vi "Vision Inspection Example (For Exe Application).vi"(4 "Thread No.":u32, 5 "ProgramRef":refnum<vi>, 6 "Thread Mod Recive":refnum<queue>[](array[refnum]), 7 "ThreadsQueue":refnum<queue>[](array[refnum]), 8 "ThreadInfoIN":T3, 10 "StackIn":cluster{"Program":i32, "Prog Index":i32}[](array[cluster]), 11 "PrameterS":string) -> (0 "ThreadInfoOUT":T3, 2 "StackOut":cluster{"Program":i32, "Prog Index":i32}[](array[cluster]), 3 "ErrorCode":string)   [LabVIEW 2020]
uses:
  <vilib>/vision/NI_Vision_Development_Module.lvlib
panel:
  in  "SettingAbort":bool
  out "P2":T1(plugin-control)
  out "P1":T1(plugin-control)
  out "Update?":bool
  in  "SettingDone":bool
  out "Result":sgl
  in  "OP Overwrite":string(combo)
  in  "SettingData":T2={"MatchParameters"={"Number of Matches Requested"=1, "Minimum Match Score"=600.0, "Angle Ranges"=[{"Start Angle"=0.0, "End Angle"=360.0}]}, "Algorithm"=1, "Pattern1ImageStriing"="", "Pattern1"={"x"=2703.5, "y"=1250.0}, "ROI"={"Global Rectangle"=[816, 381, 3234, 2692], "Contours"=[{"Contour Type"=0, "ROI Type"=3, "Points"=[816, 381, 3234, 2692]}, {"Contour Type"=0, "ROI Type"=3, "Points"=[2426, 953, 2982, 1548]}, {"Contour Type"=0, "ROI Type"=3, "Points"=[1311, 1495, 1906, 2113]}]}, "Range"={"Minimum"=160.0, "Maximum"=180.0}, "Pattern2ImageStriing"="", "Pattern2"={"x"=1608.0, "y"=1803.5}, "PatternAngle"=153.19487, "PatternImageStriing"=""} {"Pattern2"."y" format="%.2f"; "Pattern2"."x" format="%.2f"; "Range"."Maximum" format="%.2f"; "Range"."Minimum" format="%.2f"; "Pattern1"."y" format="%.2f"; "Pattern1"."x" format="%.2f"; "Algorithm" items=["All", "Low Discrepancy Sampling", "Grayscale Value Pyramid", "Gradients Pyramid"]}
  in  "ImagePath":path=path "D:/Project/Z-Other/Boash2M/sample02 cover black.png"
  out "Test":T1(plugin-control)
  out "FindPattern1?":bool
  in  "IMAQ?":bool=TRUE
  out "FindPattern2?":bool
  out "SampleAngle":sgl
  out "Pattern":T1(plugin-control)
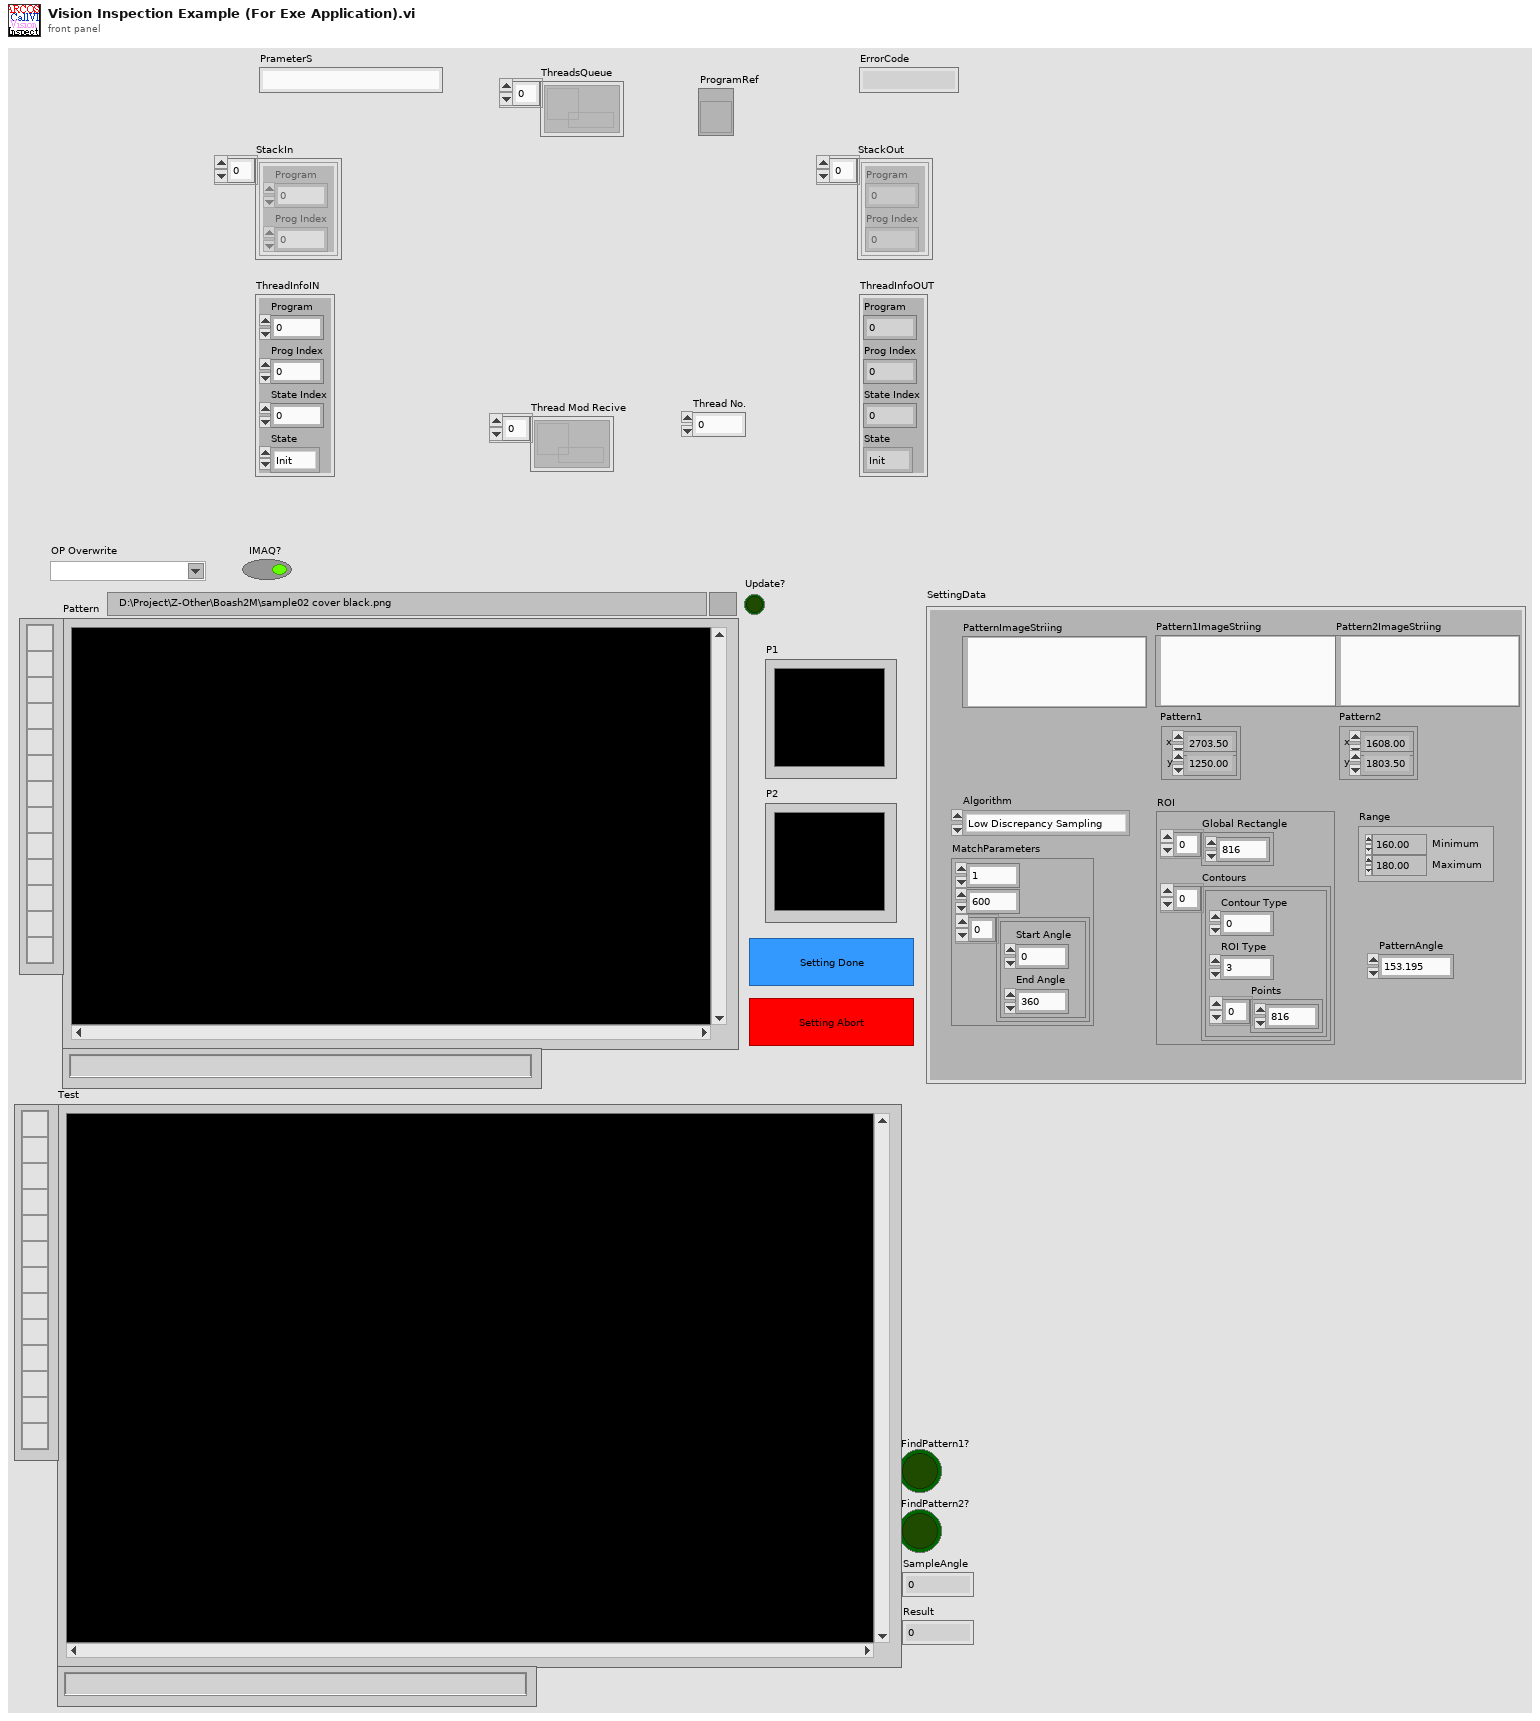
[diagram p1: front panel]
types:
  T1 = typedef "IMAQ Image.ctl" = refnum<image>
  T2 = cluster{"MatchParameters":cluster{"Number of Matches Requested":i32, "Minimum Match Score":sgl, "Angle Ranges":cluster{"Start Angle":sgl, "End Angle":sgl}[]}, "Algorithm":i32, "Pattern1ImageStriing":string, "Pattern1":cluster{"x":sgl, "y":sgl}, "ROI":cluster{"Global Rectangle":i32[], "Contours":cluster{"Contour Type":u32, "ROI Type":u32, "Points":i32[]}[]}, "Range":cluster{"Minimum":sgl, "Maximum":sgl}, "Pattern2ImageStriing":string, "Pattern2":cluster{"x":sgl, "y":sgl}, "PatternAngle":sgl, "PatternImageStriing":string}
  T3 = cluster{"Program":i32, "Prog Index":i32, "State Index":i32, "State":enum16{"Init", "Idle", "Auto Start", "Auto Running", "Step Start", "Step Running", "Suspend", "Restart", "Stop", "Reset"}}
  T4 = typedef "Image Type" = u32
  T5 = cluster{"Global Rectangle":i32[], "Contours":cluster{"Contour Type":u32, "ROI Type":u32, "Points":i32[]}[]}
  T6 = cluster{"Contour Type":u32, "ROI Type":u32, "Points":i32[]}[]
  T7 = cluster{"Contour Type":u32, "ROI Type":u32, "Points":i32[]}
  T8 = enum16{"Init", "Idle", "Auto Start", "Auto Running", "Step Start", "Step Running", "Suspend", "Restart", "Stop", "Reset"}
  T9 = cluster{"Number of Matches Requested":i32, "Minimum Match Score":sgl, "Angle Ranges":cluster{"Start Angle":sgl, "End Angle":sgl}[]}
  T10 = cluster{"Position":cluster{"x":sgl, "y":sgl}, "Angle":sgl, "Scale":sgl, "Score":sgl, "Bounding Box":cluster{"x":sgl, "y":sgl}[]}[]
  T11 = cluster{"Position":cluster{"x":sgl, "y":sgl}, "Angle":sgl, "Scale":sgl, "Score":sgl, "Bounding Box":cluster{"x":sgl, "y":sgl}[]}
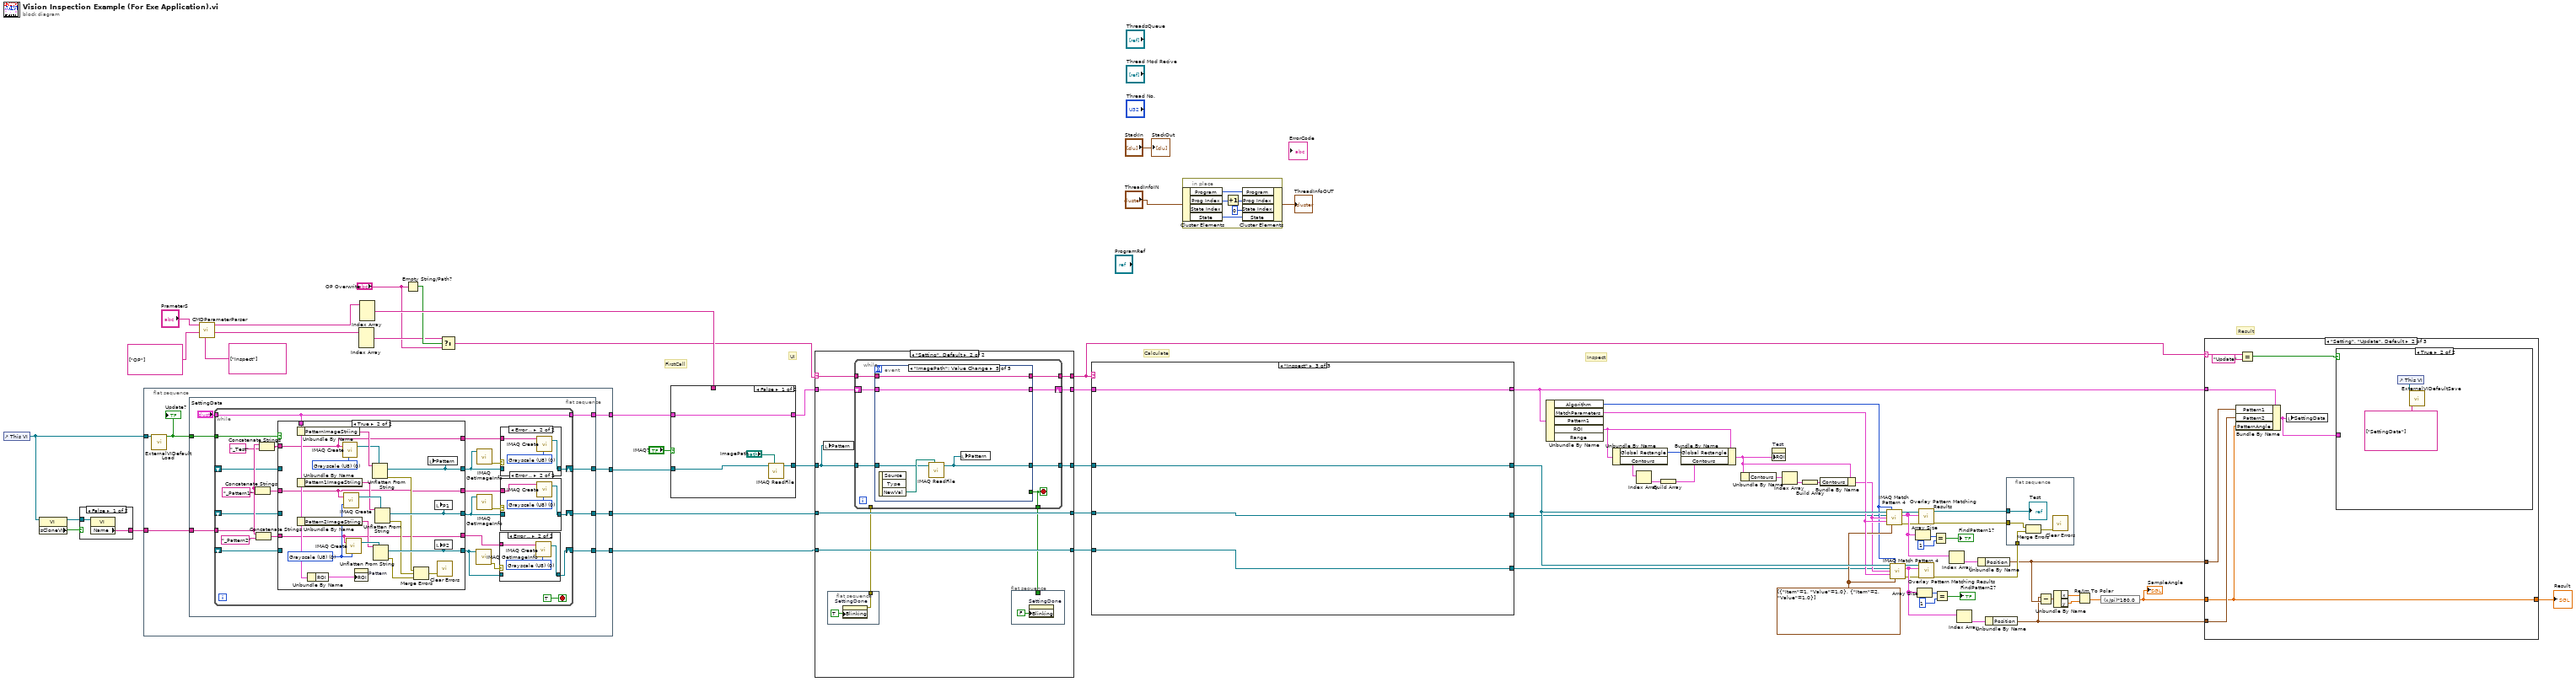
[diagram p0: block diagram]
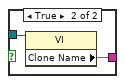
[diagram p2: hidden frame]
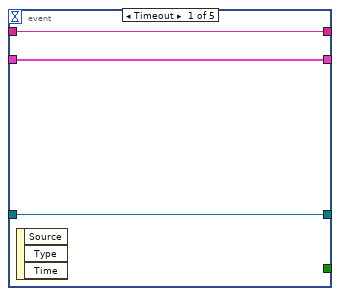
[diagram p8: hidden frame]
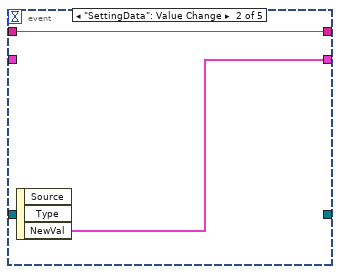
[diagram p9: hidden frame]
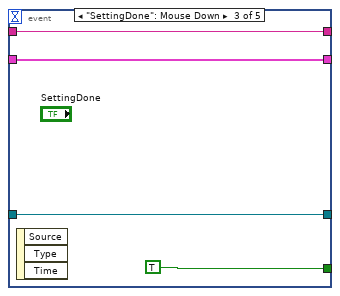
[diagram p10: hidden frame]
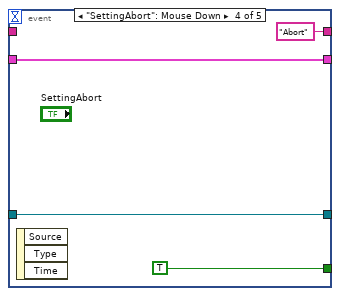
[diagram p11: hidden frame]
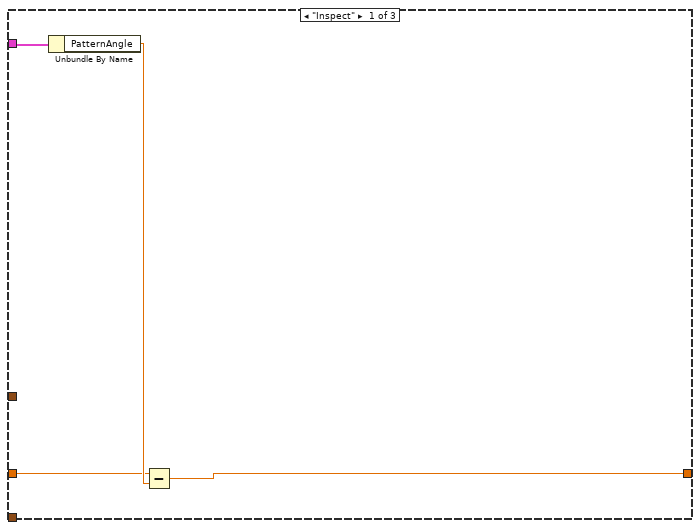
[diagram p12: hidden frame]
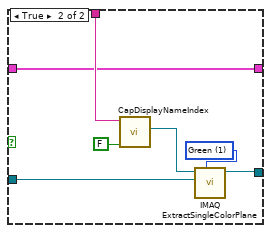
[diagram p15: hidden frame]
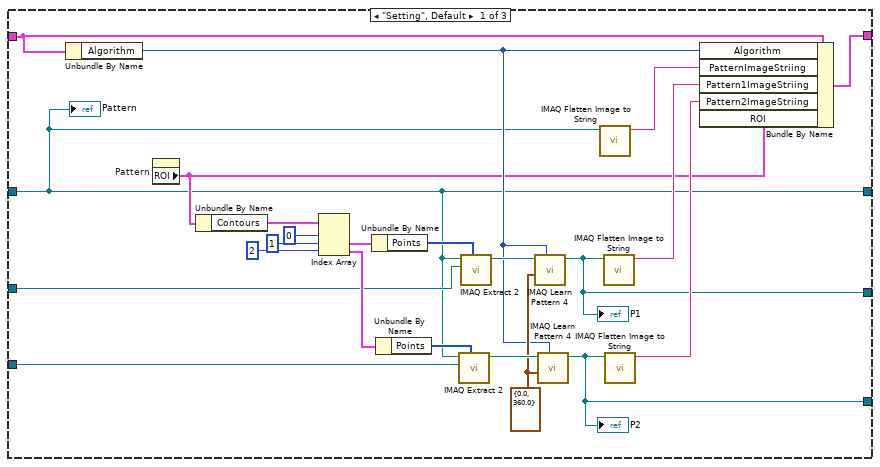
[diagram p16: hidden frame]
diagram:
  w37 = cluster{"Item":u16, "Value":dbl}[] [{"Item"=1, "Value"=1.0}, {"Item"=2, "Value"=1.0}] ("Advanced Options")
  # "Result"
  # "Inspect"
  # "Calculate"
  # "FirstCall"
  # "UI"
  n1 = control-ref of="This VI"() -> (w14:refnum<vi>)
  n2 = property class="VI"(reference=w14) -> (reference out=w15:refnum<vi>, "IsCloneVI"=w16:bool)  [unwired: 1 in, 1 out]
  n3 = case shown="False" w16 {
    tunnel: w15 -> [w73 w75]
    tunnel: [w72 w74] -> w2
    frame False {
      n4 = property class="VI"(reference=w73) -> ("Name"=w72:string)  [unwired: 1 in, 2 out]
    }
    frame True {
      n5 = property class="VI"(reference=w75) -> ("Clone Name"=w74:string)  [unwired: 1 in, 2 out]
    }
  }
  n6 = flat-sequence {
    tunnel: [w82] -> w18
    tunnel: w14 -> [w80]
    tunnel: [w77] -> w4
    tunnel: [w76] -> w3
    tunnel: w2 -> [w79]
    tunnel: [w78] -> w1
    frame #0 {
      n7 = call "ExternalVIDefaultLoad.vi"("VI in"=w80) -> ("Update?"=w81:bool)  [unwired: 10 in]
      "Update?" <- w81
      n8 = flat-sequence {
        tunnel: [w88] -> w82
        tunnel: w81 -> [w87]
        tunnel: w79 -> [w86]
        tunnel: [w85] -> w78
        tunnel: [w84] -> w77
        tunnel: [w83] -> w76
        frame #0 {
          n9 = while {
            shift-right: [w98] -> w85
            shift-left: _ -> [w111]
            shift-right: [w96] -> w84
            shift-left: _ -> [w110]
            shift-right: [w90] -> w83
            shift-left: _ -> [w109]
            tunnel: "SettingData" -> [w108]
            tunnel: [w108] -> w88
            tunnel: w87 -> [w113]
            tunnel: w86 -> [w112]
            stop <- TRUE stop-if-true
            n10 = Concatenate Strings(w112, "_Pattern1" ("string")) -> (w104:string)
            n11 = Concatenate Strings(w112, "_Pattern2" ("string")) -> (w102:string)
            n12 = Concatenate Strings(w112, "_Test" ("string")) -> (w106:string)
            n13 = case shown="True" w113 {
              tunnel: w111 -> [w130 _]
              tunnel: w110 -> [w132 _]
              tunnel: w109 -> [w131 _]
              tunnel: w108 -> [_ w145]
              tunnel: [w130 w142] -> w99
              tunnel: [w132 w141] -> w94
              tunnel: [w131 w140] -> w92
              tunnel: w106 -> [w129 w134]
              tunnel: w104 -> [w128 w135]
              tunnel: w102 -> [w127 w133]
              tunnel: [w128 w135] -> w95
              tunnel: [w129 w134] -> w100
              tunnel: [w127 w133] -> w91
              frame False {
              }
              frame True {
                w152 = T4 0 items=["Grayscale (U8)", "Grayscale (I16)", "Grayscale (SGL)", "Complex (CSG)", "RGB (U32)", "HSL (U32)", "RGB (U64)", "Grayscale (U16)"] ("Image Type")
                w143 = T4 0 items=["Grayscale (U8)", "Grayscale (I16)", "Grayscale (SGL)", "Complex (CSG)", "RGB (U32)", "HSL (U32)", "RGB (U64)", "Grayscale (U16)"] ("Image Type")
                n14 = Unbundle By Name(w145) -> ("PatternImageStriing"=w151:string)
                n15 = Unbundle By Name(w145) -> ("Pattern1ImageStriing"=w147:string)
                n16 = Unbundle By Name(w145) -> ("Pattern2ImageStriing"=w146:string)
                n17 = Unbundle By Name(w145) -> ("ROI"=w144:T5)
                n18 = call "IMAQ Create"("Image Name"=w134, "Image Type"=w152) -> ("New Image"=w150:T1)  [unwired: 3 in, 1 out]
                n19 = call "IMAQ Create"("Image Name"=w135, "Image Type"=w143) -> ("New Image"=w149:T1)  [unwired: 3 in, 1 out]
                n20 = call "IMAQ Create"("Image Name"=w133, "Image Type"=w143) -> ("New Image"=w148:T1)  [unwired: 3 in, 1 out]
                n21 = property on="Pattern" class="ImageControl"("ROI"=w144) -> ()  [unwired: 2 in, 2 out]
                n22 = Unflatten From String(type=w150, binary string=w151) -> (value=w142:T1, error out=w139:errorcluster)  [unwired: 3 in, 1 out]
                n23 = Unflatten From String(type=w148, binary string=w146) -> (value=w140:T1, error out=w137:errorcluster)  [unwired: 3 in, 1 out]
                n24 = Unflatten From String(type=w149, binary string=w147) -> (value=w141:T1, error out=w138:errorcluster)  [unwired: 3 in, 1 out]
                n25 = Merge Errors(w139, w138, w137) -> (w136:errorcluster)
                n26 = local write "Pattern"(w142) -> ()
                n27 = local write "P1"(w141) -> ()
                n28 = local write "P2"(w140) -> ()
                n29 = call <vilib>:"Clear Errors.vi"("error in (no error)"=w136) -> ()  [unwired: 5 in, 2 out]
              }
            }
            n30 = call "IMAQ GetImageInfo"("Image"=w92) -> ("error out"=w93:errorcluster)  [unwired: 3 in, 7 out]
            n31 = call "IMAQ GetImageInfo"("Image"=w99) -> ("error out"=w101:errorcluster)  [unwired: 3 in, 7 out]
            n32 = call "IMAQ GetImageInfo"("Image"=w94) -> ("error out"=w97:errorcluster)  [unwired: 3 in, 7 out]
            n33 = case shown="Error .." w93 {
              tunnel: w91 -> [_ w118]
              tunnel: w92 -> [w115 _]
              tunnel: [w115 w116] -> w90
              frame No Error {
              }
              frame Error {
                w117 = T4 0 items=["Grayscale (U8)", "Grayscale (I16)", "Grayscale (SGL)", "Complex (CSG)", "RGB (U32)", "HSL (U32)", "RGB (U64)", "Grayscale (U16)"] ("Image Type")
                n34 = call "IMAQ Create"("Image Name"=w118, "Image Type"=w117) -> ("New Image"=w116:T1)  [unwired: 3 in, 1 out]
              }
            }
            n35 = case shown="Error .." w101 {
              tunnel: w100 -> [_ w126]
              tunnel: w99 -> [w123 _]
              tunnel: [w123 w124] -> w98
              frame No Error {
              }
              frame Error {
                w125 = T4 0 items=["Grayscale (U8)", "Grayscale (I16)", "Grayscale (SGL)", "Complex (CSG)", "RGB (U32)", "HSL (U32)", "RGB (U64)", "Grayscale (U16)"] ("Image Type")
                n36 = call "IMAQ Create"("Image Name"=w126, "Image Type"=w125) -> ("New Image"=w124:T1)  [unwired: 3 in, 1 out]
              }
            }
            n37 = case shown="Error .." w97 {
              tunnel: w94 -> [w119 _]
              tunnel: [w119 w121] -> w96
              tunnel: w95 -> [_ w120]
              frame No Error {
              }
              frame Error {
                w122 = T4 0 items=["Grayscale (U8)", "Grayscale (I16)", "Grayscale (SGL)", "Complex (CSG)", "RGB (U32)", "HSL (U32)", "RGB (U64)", "Grayscale (U16)"] ("Image Type")
                n38 = call "IMAQ Create"("Image Name"=w120, "Image Type"=w122) -> ("New Image"=w121:T1)  [unwired: 3 in, 1 out]
              }
            }
          }
        }
      }
    }
  }
  n39 = call "CMDParameterParser.vi"("DeafultValues"=string[] ["Inspect"], "RequiredKeys"=string[] ["OP"], "CMDParameter"="PrameterS") -> ("KeyValues"=w67:string[], "Input"=w65:string[])  [unwired: 6 in, 1 out]
  n40 = Index Array(array=w67) -> (element #1=w29:string)  [unwired: 3 in, 2 out]
  n41 = Index Array(array=w65) -> (element #1=w64:string)  [unwired: 3 in, 2 out]
  n42 = Empty String/Path?(string/path="OP Overwrite") -> (empty?=w30:bool)
  n43 = Select(t=w29, s=w30, f="OP Overwrite") -> (s? t:f=w13:string)
  n44 = case shown="False" "IMAQ?" {
    tunnel: [w156 w159] -> w19
    tunnel: w64 -> [_ w162]
    tunnel: w1 -> [w154 w158]
    tunnel: w18 -> [w153 w157]
    tunnel: [w153 w157] -> w17
    frame False {
      n45 = call "IMAQ ReadFile"("File Path"="ImagePath", "Image"=w154) -> ("Image Out"=w156:T1)  [unwired: 5 in, 4 out]
    }
    frame True {
      w161 = 1 items=["Red", "Green", "Blue", "Hue", "Saturation", "Luminance", "Value", "Intensity"] ("Color Plane")
      n46 = call "CapDisplayNameIndex.vi"("Init?"=FALSE, "CamName"=w162) -> ("IMAQ"=w160:T1)  [unwired: 3 in, 3 out]
      n47 = call "IMAQ ExtractSingleColorPlane"("Color Plane"=w161, "Image Dst"=w158, "Image Src"=w160) -> ("Image Dst Out"=w159:T1)  [unwired: 7 in, 1 out]
    }
  }
  n48 = case shown="\"Setting\", Default" w13 {
    selector: w13 -> [w164 w171]
    tunnel: w17 -> [w168 w175]
    tunnel: [w168 w174] -> w22
    tunnel: w19 -> [w167 w169]
    tunnel: [w167 w176] -> w21
    tunnel: w4 -> [w166 w178]
    tunnel: [w166 w178] -> w20
    tunnel: w3 -> [w165 w177]
    tunnel: [w165 w177] -> w9
    tunnel: [w164 w170] -> w12
    frame "Inspect" {
    }
    frame "Setting", Default {
      n49 = local write "Pattern"(w169) -> ()
      n50 = flat-sequence {
        tunnel: [w180] -> w173
        frame #0 {
          n51 = property on="SettingDone" class="Bool"("Blinking"=TRUE) -> (error out=w180:errorcluster)  [unwired: 2 in, 1 out]
        }
      }
      n52 = while {
        tunnel: w169 -> [w188]
        tunnel: [w187] -> w176
        shift-right: [w186] -> w174
        shift-left: w175 -> [w185]
        tunnel: w173 -> [_]
        tunnel: [w184] -> w172
        tunnel: w171 -> [w183]
        tunnel: [w182] -> w170
        stop <- w184 stop-if-true
        n53 = event shown="[4] \"ImagePath\": Value Change" {
          selector: _ -> [_ _ _ _ _]
          dyn-events: _ -> [_ _ _ _ _]
          timeout: _ -> [_ _ _ _ _]
          tunnel: [_ _ TRUE TRUE _] -> w184
          tunnel: w188 -> [w191 _ w196 w200 w205]
          tunnel: [w191 _ w196 w200 w203] -> w187
          tunnel: [w189 w193 w195 w199 w204] -> w186
          tunnel: w185 -> [w189 _ w195 w199 w204]
          tunnel: w183 -> [w190 w192 w194 _ w202]
          tunnel: [w190 w192 w194 "Abort" w202] -> w182
          event Timeout {
            n54 = event-data() -> ()  [unwired: 1 in, 3 out]
          }
          event "SettingData": Value Change {
            n55 = event-data() -> ("NewVal"=w193:T2)  [unwired: 1 in, 2 out]
          }
          event "SettingDone": Mouse Down {
            n56 = event-data() -> ()  [unwired: 1 in, 3 out]
          }
          event "SettingAbort": Mouse Down {
            n57 = event-data() -> ()  [unwired: 1 in, 3 out]
          }
          event "ImagePath": Value Change {
            n58 = event-data() -> ("NewVal"=w206:path)  [unwired: 1 in, 2 out]
            n59 = call "IMAQ ReadFile"("File Path"=w206, "Image"=w205) -> ("Image Out"=w203:T1)  [unwired: 5 in, 4 out]
            n60 = local write "Pattern"(w203) -> ()
          }
        }
      }
      n61 = flat-sequence {
        tunnel: w172 -> [_]
        frame #0 {
          n62 = property on="SettingDone" class="Bool"("Blinking"=FALSE) -> ()  [unwired: 2 in, 2 out]
        }
      }
    }
  }
  n63 = case shown="\"Inspect\"" w12 {
    tunnel: w22 -> [w215 w233 w236]
    tunnel: w21 -> [w208 w232 w237]
    tunnel: [w214 w233 w236] -> w31
    tunnel: [w210 w231 w235] -> w6
    tunnel: [w209 w230 w234] -> w5
    tunnel: [w208 w232 w237] -> w39
    tunnel: w9 -> [w211 w230 w234]
    tunnel: w20 -> [w212 w231 w235]
    frame "Setting", Default {
      w218 = cluster{"Start Angle":sgl, "End Angle":sgl} {"Start Angle"=0.0, "End Angle"=360.0} ("Angle Range")
      n64 = Unbundle By Name(w215) -> ("Algorithm"=w216:i32)
      n65 = property on="Pattern" class="ImageControl"() -> ("ROI"=w213:T5)  [unwired: 2 in, 2 out]
      n66 = Unbundle By Name(w213) -> ("Contours"=w228:T6)
      n67 = Index Array(array=w228, index #1=0 ("index"), index #2=1 ("index"), index #3=2 ("index")) -> (element #2=w223:T7, element #3=w220:T7)  [unwired: 1 out]
      n68 = Unbundle By Name(w223) -> ("Points"=w222:i32[])
      n69 = Unbundle By Name(w220) -> ("Points"=w221:i32[])
      n70 = call "IMAQ Extract 2"("Optional Rectangle"=w221, "Image Dst"=w211, "Image Src"=w208) -> ("Image Dst Out"=w219:T1)  [unwired: 7 in, 1 out]
      n71 = call "IMAQ Extract 2"("Optional Rectangle"=w222, "Image Dst"=w212, "Image Src"=w208) -> ("Image Dst Out"=w226:T1)  [unwired: 7 in, 1 out]
      n72 = call "IMAQ Learn Pattern 4"("Algorithm"=w216, "Angle Range"=w218, "Image"=w226) -> ("Template Image Out"=w210:T1)  [unwired: 6 in, 2 out]
      "P1" <- w210
      n73 = call "IMAQ Learn Pattern 4"("Algorithm"=w216, "Angle Range"=w218, "Image"=w219) -> ("Template Image Out"=w209:T1)  [unwired: 6 in, 2 out]
      "P2" <- w209
      n74 = call "IMAQ Flatten Image to String"("Image"=w208) -> ("Data String"=w207:string)  [unwired: 9 in, 1 out]
      n75 = call "IMAQ Flatten Image to String"("Image"=w210) -> ("Data String"=w229:string)  [unwired: 9 in, 1 out]
      n76 = call "IMAQ Flatten Image to String"("Image"=w209) -> ("Data String"=w217:string)  [unwired: 9 in, 1 out]
      n77 = Bundle By Name(cluster=w215, "Algorithm"=w216, "PatternImageStriing"=w207, "Pattern1ImageStriing"=w229, "Pattern2ImageStriing"=w217, "ROI"=w213) -> (w214:T2)
      "Pattern" <- w208
    }
    frame "Abort" {
    }
    frame "Inspect" {
    }
  }
  n78 = in-place {
    n79 = in-place-cluster #1("ThreadInfoIN") -> ("Program"=w242:i32, "Prog Index"=w240:i32, "State"=w238:T8)  [unwired: 1 out]
    n80 = Increment(x=w240) -> (x+1=w241:i32)
    n81 = in-place-cluster #1("Program"=w242, "Prog Index"=w241, "State Index"=0, "State"=w238) -> (→"ThreadInfoOUT":T3)
  }
  n82 = Unbundle By Name(w31) -> ("Algorithm"=w32:i32, "MatchParameters"=w38:T9, "ROI"=w48:T5)  [unwired: 2 out]
  n83 = Unbundle By Name(w48) -> ("Global Rectangle"=w47:i32[], "Contours"=w44:T6)
  n84 = Index Array(array=w44) -> (element=w45:T7)  [unwired: 1 in]
  n85 = Build Array(w45) -> (w46:T6)
  n86 = Bundle By Name(cluster=w48, "Global Rectangle"=w47, "Contours"=w46) -> (w40:T5)
  n87 = Unbundle By Name(w40) -> ("Contours"=w50:T6)
  n88 = property on="Test" class="ImageControl"("ROI"=w40) -> ()  [unwired: 2 in, 2 out]
  n89 = Index Array(array=w50) -> (element=w51:T7)  [unwired: 1 in]
  n90 = Build Array(w51) -> (w52:T6)
  n91 = Bundle By Name(cluster=w40, "Contours"=w52) -> (w33:T5)
  n92 = call "IMAQ Match Pattern 4"("Image"=w39, "Algorithm"=w32, "Template Image"=w6, "ROI Descriptor"=w33, "Parameters"=w38, "Advanced Options"=w37) -> ("Image (duplicate)"=w49:T1, "Matches (pixel)"=w58:T10, "error out"=w11:errorcluster)  [unwired: 5 in, 2 out]
  n93 = call "IMAQ Match Pattern 4"("Image"=w39, "Algorithm"=w32, "Template Image"=w5, "ROI Descriptor"=w33, "Parameters"=w38, "Advanced Options"=w37) -> ("Image (duplicate)"=w53:T1, "Matches (pixel)"=w34:T10, "error out"=w10:errorcluster)  [unwired: 5 in, 2 out]
  n94 = Array Size(array=w58) -> (size(s)=w43:i32)
  n95 = Array Size(array=w34) -> (size(s)=w54:i32)
  n96 = call "Overlay Pattern Matching Results.vi"("error in"=w11, "Matches"=w58, "Image"=w49) -> ("error out"=w36:errorcluster, "Image Out"=w7:T1)  [unwired: 7 in]
  n97 = call "Overlay Pattern Matching Results.vi"("error in"=w10, "Matches"=w34, "Image"=w53) -> ("error out"=w35:errorcluster)  [unwired: 7 in, 1 out]
  n98 = Equal?(x=w43, y=1) -> (x = y?=→"FindPattern1?":bool)
  n99 = Equal?(x=w54, y=1) -> (x = y?=→"FindPattern2?":bool)
  n100 = Index Array(array=w58) -> (element=w57:T11)  [unwired: 1 in]
  n101 = Index Array(array=w34) -> (element=w59:T11)  [unwired: 1 in]
  n102 = Unbundle By Name(w57) -> ("Position"=w25:cluster{"x":sgl, "y":sgl})
  n103 = Unbundle By Name(w59) -> ("Position"=w24:cluster{"x":sgl, "y":sgl})
  n104 = flat-sequence {
    tunnel: w36 -> [w245]
    tunnel: w35 -> [w244]
    tunnel: w7 -> [w246]
    frame #0 {
      n105 = Merge Errors(w245, w244) -> (w243:errorcluster)
      n106 = call <vilib>:"Clear Errors.vi"("error in (no error)"=w243) -> ()  [unwired: 5 in, 2 out]
      "Test" <- w246
    }
  }
  n107 = Subtract(x=w24, y=w25) -> (x-y=w60:cluster{"x":sgl, "y":sgl})
  n108 = Unbundle By Name(w60) -> ("x"=w61:sgl, "y"=w62:sgl)
  n109 = Re/Im To Polar(2:w62, 3:w61) -> (0:w63:sgl)  [unwired: 1 out]
  n110 = expression code="(x/pi)*180.0" ("radians to degrees")(w63) -> (w8:sgl)
  "SampleAngle" <- w8
  n111 = case shown="\"Setting\", \"Update\", Default" w12 {
    selector: w12 -> [_ w254 _]
    tunnel: w25 -> [_ w257 _]
    tunnel: w24 -> [_ w256 _]
    tunnel: w31 -> [w250 w258 _]
    tunnel: w8 -> [w248 w255 _]
    tunnel: [w247 w255 _] -> w23
    frame "Inspect" {
      n112 = Unbundle By Name(w250) -> ("PatternAngle"=w249:sgl)
      n113 = Subtract(x=w248, y=w249) -> (x-y=w247:sgl)
    }
    frame "Setting", "Update", Default {
      n114 = Bundle By Name(cluster=w258, "Pattern1"=w257, "Pattern2"=w256, "PatternAngle"=w255) -> (w251:T2)
      n115 = Equal?(x=w254, y="Update") -> (x = y?=w252:bool)
      n116 = local write "SettingData"(w251) -> ()
      n117 = case shown="True" w252 {
        tunnel: w251 -> [_ _]
        frame False {
        }
        frame True {
          n118 = control-ref of="This VI"() -> (w260:refnum<vi>)
          n119 = call "ExternalVIDefaultSave.vi"("Control2SetDefault"=string[] ["SettingData"], "VI in"=w260) -> ()  [unwired: 10 in]
        }
      }
    }
    frame "Abort" {
    }
  }
  "Result" <- w23
  "StackOut" <- "StackIn"
